vi "SaveLoadControlValues.vi"(7 "Dat file (empty)":path, 8 "error in (no error)":errorcluster, 9 "Specific controls/indicators":string[](array[string]), 10 "Controls or indicators?":T1(ring), 11 "Function (Load)":enum16{"Load", "Save"}(ring)) -> (0 "error out":errorcluster)   [LabVIEW 2015]
doc: "Use this as a SubVI inside a VI that you want to save and load the controls/indicators from. Refer to the <B>SaveLoadControlValuesDemo.vi</B> to see a demonstration of how to use this VI.\n\n<B>Dat file</B> specifies the name and path of the *.dat file. If the control is empty, the default file will be used (see block diagram for further information).\n\nIf names are specified in <B>Specific controls/indicators</B>, the <B>Controls or indicators?</B> will be ignored."
panel:
  # "Use this as a SubVI inside a VI that you want to save and load the controls/indicators from. Refer to the \"SaveLoadControlValuesDemo.vi\" to see a demonstration of how to use this VI.\n\nFor more information, see the block diagram or go to\nFile >> VI Properties... >> Documentation"
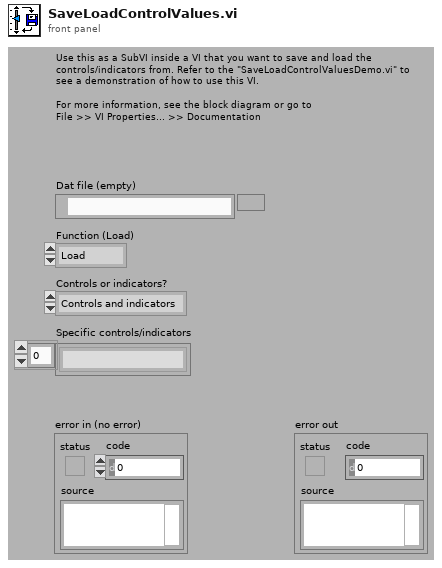
[diagram p1: front panel]
types:
  T1 = enum16{"Controls and indicators", "Controls only", "Indicators only"}
  T2 = enum16{"open", "replace", "create", "open or create", "replace or create", "replace or create with confirmation"}
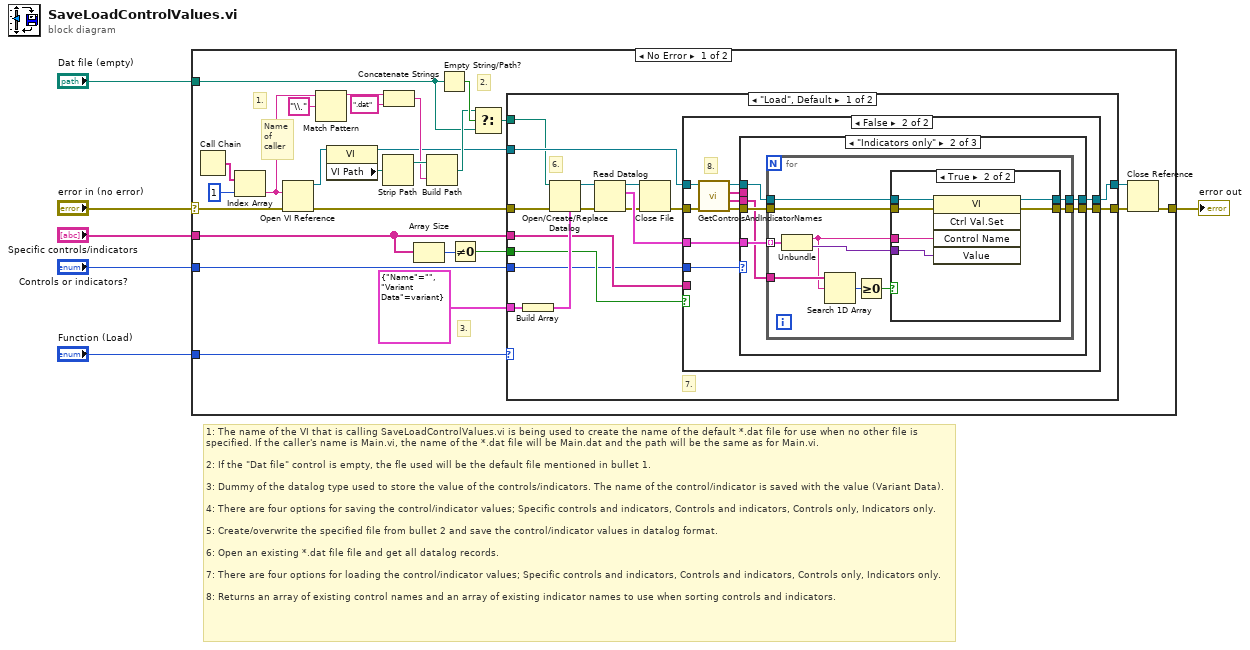
[diagram p0: block diagram]
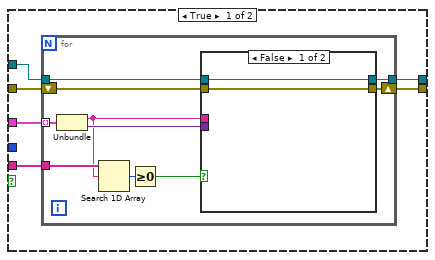
[diagram p2: hidden frame]
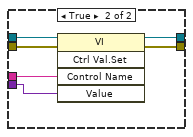
[diagram p3: hidden frame]
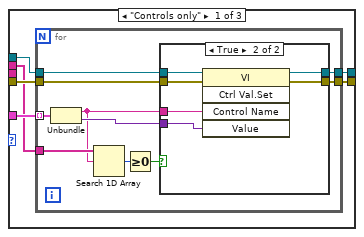
[diagram p4: hidden frame]
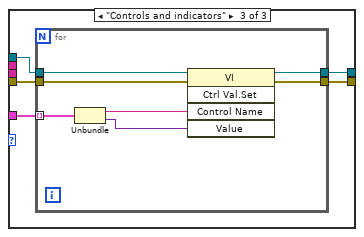
[diagram p7: hidden frame]
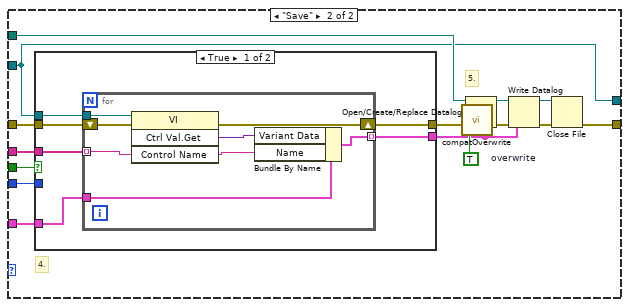
[diagram p8: hidden frame]
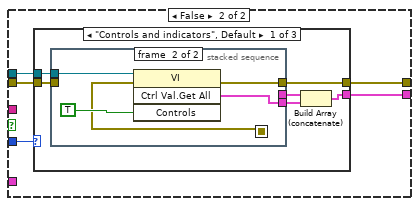
[diagram p9: hidden frame]
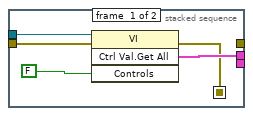
[diagram p10: hidden frame]
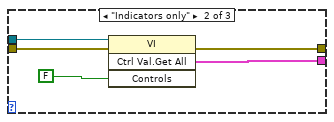
[diagram p11: hidden frame]
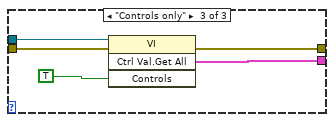
[diagram p12: hidden frame]
diagram:
  # "1: The name of the VI that is calling SaveLoadControlValues.vi is being used to create the name of the default *.dat file for use when no other file is specified. If the caller's name is Main.vi, the name of the *.dat file will be Main.dat and the path will be the same as for Main.vi.\n\n2: If the \"Dat file\" control is empty, the fle used will be the default file mentioned in bullet 1.\n\n3: Dummy of the datalog type used to store the value of the controls/indicators. The name of the control/indicator is saved with the value (Variant Data).\n\n4: There are four options for saving the control/indicator values; Specific controls and indicators, Controls and indicators, Controls only, Indicators only.\n\n5: Create/overwrite the specified file from bullet 2 and save the control/indicator values in datalog format.\n\n6: Open an existing *.dat file file and get all datalog records.\n\n7: There are four options for loading the control/indicator values; Specific controls and indicators, Controls and indicators, Controls only, Indicators only.\n\n8: Returns an array of existing control names and an array of existing indicator names to use when sorting controls and indicators."
  n1 = case shown="No Error" "error in (no error)" {
    selector: "error in (no error)" -> [w25 w203]
    tunnel: [w27 w203] -> w6
    tunnel: "Dat file (empty)" -> [w14 _]
    tunnel: "Function (Load)" -> [w13 _]
    tunnel: "Controls or indicators?" -> [w9 _]
    tunnel: "Specific controls/indicators" -> [w8 _]
    frame No Error {
      # "3."
      # "2."
      # "1."
      # "Name of caller"
      n2 = Call Chain() -> (call chain=w32:string[])
      n3 = Index Array(array=w32, index=1) -> (element=w19:string)
      n4 = Open VI Reference(vi path=w19, error in (no error)=w25) -> (vi reference=w23:refnum<vi>, error out=w30:errorcluster)  [unwired: 4 in]
      n5 = Match Pattern(string=w19, regular expression="\\.") -> (before substring=w18:string)  [unwired: 1 in, 3 out]
      n6 = property class="VI"(reference=w23) -> (reference out=w7:refnum<vi>, "VI Path"=w22:path)  [unwired: 1 in, 1 out]
      n7 = Strip Path(path=w22) -> (stripped path=w26:path)  [unwired: 1 out]
      n8 = Concatenate Strings(w18, ".dat" ("Name of ini file 2")) -> (w17:string)
      n9 = Array Size(array=w8) -> (size(s)=w12:i32)
      n10 = Build Path(base path=w26, name or relative path=w17) -> (appended path=w16:path)
      n11 = Empty String/Path?(string/path=w14) -> (empty?=w24:bool)
      n12 = Not Equal To 0?(x=w12) -> (x != 0?=w11:bool)
      n13 = Select(t=w16, s=w24, f=w14) -> (s? t:f=w15:path)
      n14 = case shown="\"Load\", Default" w13 {
        tunnel: w15 -> [w41 w153]
        tunnel: w7 -> [w45 w152]
        tunnel: w30 -> [w44 w154]
        tunnel: [w43 w152] -> w29
        tunnel: [w42 w145] -> w28
        tunnel: w11 -> [w37 w151]
        tunnel: w8 -> [w38 w150]
        tunnel: cluster{"Name":string, "Variant Data":variant} {"Name"="", "Variant Data"=variant} -> [w40 w148]
        tunnel: w9 -> [w33 w147]
        frame "Load", Default {
          # "7."
          # "6."
          n15 = Build Array(w40) -> (w39:cluster{"Name":string, "Variant Data":variant}[])
          n16 = Open/Create/Replace Datalog(5:w39, 8:w44, 11:w41) -> (0:w46:errorcluster, 3:w47:refnum<k1>)  [unwired: 3 in, 1 out]
          n17 = Read Datalog(4:w46, 7:w47) -> (0:w36:errorcluster, 2:w48:cluster{"Name":string, "Variant Data":variant}[], 3:w34:refnum<k1>)  [unwired: 1 in]
          n18 = Close File(refnum=w34, error in=w36) -> (error out=w35:errorcluster)  [unwired: 1 out]
          n19 = case shown="False" w37 {
            tunnel: w48 -> [w54 w82]
            tunnel: w45 -> [w53 w79]
            tunnel: w35 -> [w52 w78]
            tunnel: [w51 w81] -> w43
            tunnel: [w50 w80] -> w42
            tunnel: w38 -> [w49 _]
            tunnel: w33 -> [_ w75]
            frame True {
              n20 = for {
                tunnel: w54 -> [w58] mode=indexing
                tunnel: w53 -> [w63]
                tunnel: [w60] -> w51
                tunnel: w49 -> [w59]
                shift-right: [w61] -> w50
                shift-left: w52 -> [w62]
                n21 = Unbundle(w58) -> ("Name"=w57:string, "Variant Data"=w64:variant)
                n22 = Search 1D Array(1D array=w59, element=w57) -> (index of element=w56:i32)  [unwired: 1 in]
                n23 = Greater Or Equal To 0?(x=w56) -> (x >= 0?=w55:bool)
                n24 = case shown="False" w55 {
                  tunnel: w64 -> [_ w72]
                  tunnel: w63 -> [w65 w71]
                  tunnel: w62 -> [w66 w70]
                  tunnel: [w66 w69] -> w61
                  tunnel: [w65 w68] -> w60
                  tunnel: w57 -> [_ w67]
                  frame False {
                  }
                  frame True {
                    n25 = invoke class="VI" method="Ctrl Val.Set"(reference=w71, error in=w70, "Control Name"=w67, "Value"=w72) -> (reference out=w68:refnum<vi>, error out=w69:errorcluster)  [unwired: 1 in, 3 out]
                  }
                }
              }
            }
            frame False {
              # "8."
              n26 = call "GetControlsAndIndicatorNames.vi"("error in (no error)"=w78, "VI Refnum"=w79) -> ("error out"=w76:errorcluster, "Indicators"=w73:string[], "Controls"=w74:string[], "VI Refnum out"=w77:refnum<vi>)  [unwired: 6 in]
              n27 = case shown="\"Indicators only\"" w75 {
                tunnel: w82 -> [w88 w112 w135]
                tunnel: [w87 w111 w134] -> w81
                tunnel: [w86 w110 w133] -> w80
                tunnel: w77 -> [w85 w109 w132]
                tunnel: w76 -> [w84 w108 w131]
                tunnel: w74 -> [w83 _ _]
                tunnel: w73 -> [_ w107 _]
                frame "Controls only" {
                  n28 = for {
                    tunnel: w88 -> [w93] mode=indexing
                    tunnel: w85 -> [w97]
                    tunnel: w84 -> [w96]
                    tunnel: [w95] -> w86
                    tunnel: [w94] -> w87
                    tunnel: w83 -> [w91]
                    n29 = Unbundle(w93) -> ("Name"=w90:string, "Variant Data"=w98:variant)
                    n30 = Search 1D Array(1D array=w91, element=w90) -> (index of element=w92:i32)  [unwired: 1 in]
                    n31 = Greater Or Equal To 0?(x=w92) -> (x >= 0?=w89:bool)
                    n32 = case shown="True" w89 {
                      tunnel: w98 -> [_ w106]
                      tunnel: w97 -> [w100 w105]
                      tunnel: w96 -> [w99 w104]
                      tunnel: [w99 w103] -> w95
                      tunnel: [w100 w102] -> w94
                      tunnel: w90 -> [_ w101]
                      frame False {
                      }
                      frame True {
                        n33 = invoke class="VI" method="Ctrl Val.Set"(reference=w105, error in=w104, "Control Name"=w101, "Value"=w106) -> (reference out=w102:refnum<vi>, error out=w103:errorcluster)  [unwired: 1 in, 3 out]
                      }
                    }
                  }
                }
                frame "Indicators only" {
                  n34 = for {
                    tunnel: w112 -> [w117] mode=indexing
                    tunnel: w109 -> [w121]
                    tunnel: w108 -> [w120]
                    tunnel: [w119] -> w110
                    tunnel: [w118] -> w111
                    tunnel: w107 -> [w115]
                    n35 = Unbundle(w117) -> ("Name"=w114:string, "Variant Data"=w122:variant)
                    n36 = Search 1D Array(1D array=w115, element=w114) -> (index of element=w116:i32)  [unwired: 1 in]
                    n37 = Greater Or Equal To 0?(x=w116) -> (x >= 0?=w113:bool)
                    n38 = case shown="True" w113 {
                      tunnel: w122 -> [_ w130]
                      tunnel: w121 -> [w124 w129]
                      tunnel: w120 -> [w123 w128]
                      tunnel: [w123 w127] -> w119
                      tunnel: [w124 w126] -> w118
                      tunnel: w114 -> [_ w125]
                      frame False {
                      }
                      frame True {
                        n39 = invoke class="VI" method="Ctrl Val.Set"(reference=w129, error in=w128, "Control Name"=w125, "Value"=w130) -> (reference out=w126:refnum<vi>, error out=w127:errorcluster)  [unwired: 1 in, 3 out]
                      }
                    }
                  }
                }
                frame "Controls and indicators" {
                  n40 = for {
                    tunnel: w135 -> [w137] mode=indexing
                    tunnel: w132 -> [w141]
                    tunnel: w131 -> [w140]
                    tunnel: [w139] -> w133
                    tunnel: [w138] -> w134
                    n41 = Unbundle(w137) -> ("Name"=w136:string, "Variant Data"=w142:variant)
                    n42 = invoke class="VI" method="Ctrl Val.Set"(reference=w141, error in=w140, "Control Name"=w136, "Value"=w142) -> (reference out=w138:refnum<vi>, error out=w139:errorcluster)  [unwired: 1 in, 3 out]
                  }
                }
              }
            }
          }
        }
        frame "Save" {
          w158 = TRUE  # overwrite
          # "5."
          # "4."
          n43 = case shown="True" w151 {
            tunnel: [w161 w172] -> w149
            tunnel: [w160 w176] -> w155
            tunnel: w154 -> [w164 w175]
            tunnel: w152 -> [w163 w174]
            tunnel: w150 -> [w162 _]
            tunnel: w148 -> [w159 _]
            tunnel: w147 -> [_ w173]
            frame True {
              n44 = for {
                tunnel: w163 -> [w170]
                tunnel: w162 -> [w168] mode=indexing
                tunnel: [w167] -> w161 mode=indexing
                tunnel: w159 -> [w165]
                shift-right: [w166] -> w160
                shift-left: w164 -> [w171]
                n45 = invoke class="VI" method="Ctrl Val.Get"(reference=w170, error in=w171, "Control Name"=w168) -> (error out=w166:errorcluster, "Get Control Value Variant"=w169:variant)  [unwired: 1 in, 2 out]
                n46 = Bundle By Name(cluster=w165, "Variant Data"=w169, "Name"=w168) -> (w167:cluster{"Name":string, "Variant Data":variant})
              }
            }
            frame False {
              n47 = case shown="\"Controls and indicators\", Default" w173 {
                tunnel: [w182 w193 w202] -> w176
                tunnel: w175 -> [w181 w197 w199]
                tunnel: w174 -> [w180 w196 w201]
                tunnel: [w177 w195 w198] -> w172
                frame "Controls and indicators", Default {
                  n48 = stacked-sequence {
                    seq-local: [w183 _] -> [_ w188]
                    tunnel: w180 -> [w187 w192]
                    tunnel: [w186 _] -> w178
                    tunnel: [_ w190] -> w179
                    tunnel: [_ w189] -> w182
                    tunnel: w181 -> [w184 _]
                    frame #0 {
                      n49 = invoke class="VI" method="Ctrl Val.Get All"(reference=w187, error in=w184, "Controls"=FALSE) -> (error out=w183:errorcluster, "Get All Control Values Variant"=w186:cluster{"Name":string, "Variant Data":variant}[])  [unwired: 1 in, 2 out]
                    }
                    frame #1 {
                      n50 = invoke class="VI" method="Ctrl Val.Get All"(reference=w192, error in=w188, "Controls"=TRUE) -> (error out=w189:errorcluster, "Get All Control Values Variant"=w190:cluster{"Name":string, "Variant Data":variant}[])  [unwired: 1 in, 2 out]
                    }
                  }
                  n51 = Build Array (concatenate)(w178, w179) -> (w177:cluster{"Name":string, "Variant Data":variant}[])
                }
                frame "Indicators only" {
                  n52 = invoke class="VI" method="Ctrl Val.Get All"(reference=w196, error in=w197, "Controls"=FALSE) -> (error out=w193:errorcluster, "Get All Control Values Variant"=w195:cluster{"Name":string, "Variant Data":variant}[])  [unwired: 1 in, 2 out]
                }
                frame "Controls only" {
                  n53 = invoke class="VI" method="Ctrl Val.Get All"(reference=w201, error in=w199, "Controls"=TRUE) -> (error out=w202:errorcluster, "Get All Control Values Variant"=w198:cluster{"Name":string, "Variant Data":variant}[])  [unwired: 1 in, 2 out]
                }
              }
            }
          }
          n54 = call <vilib>:"compatOverwrite.vi"("overwrite (F)"=w158) -> ("overwrite?"=w143:T2)
          n55 = Open/Create/Replace Datalog(5:w149, 8:w155, 10:w143, 11:w153) -> (0:w156:errorcluster, 3:w157:refnum<k1>)  [unwired: 2 in, 1 out]
          n56 = Write Datalog(4:w156, 6:w149, 7:w157) -> (0:w146:errorcluster, 3:w144:refnum<k1>)
          n57 = Close File(refnum=w144, error in=w146) -> (error out=w145:errorcluster)  [unwired: 1 out]
        }
      }
      n58 = Close Reference(reference=w29, error in (no error)=w28) -> (error out=w27:errorcluster)
    }
    frame Error {
    }
  }
  "error out" <- w6
